vi "TEST_NT_HELPER_INT.vi"() -> ()   [LabVIEW 2023]
uses:
  <vilib>/Rock Robotics/Network Tables/NT Read Integer.vi
  <vilib>/Rock Robotics/Network Tables/NT Write Integer.vi
panel:
  out "value 2":i64
  out "value":i64
  in  "name 2":string="Test4150Val1i"
  in  "name":string="Test4150Val2i"
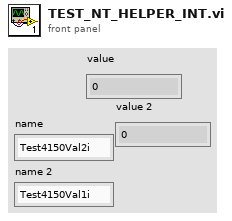
[diagram p1: front panel]
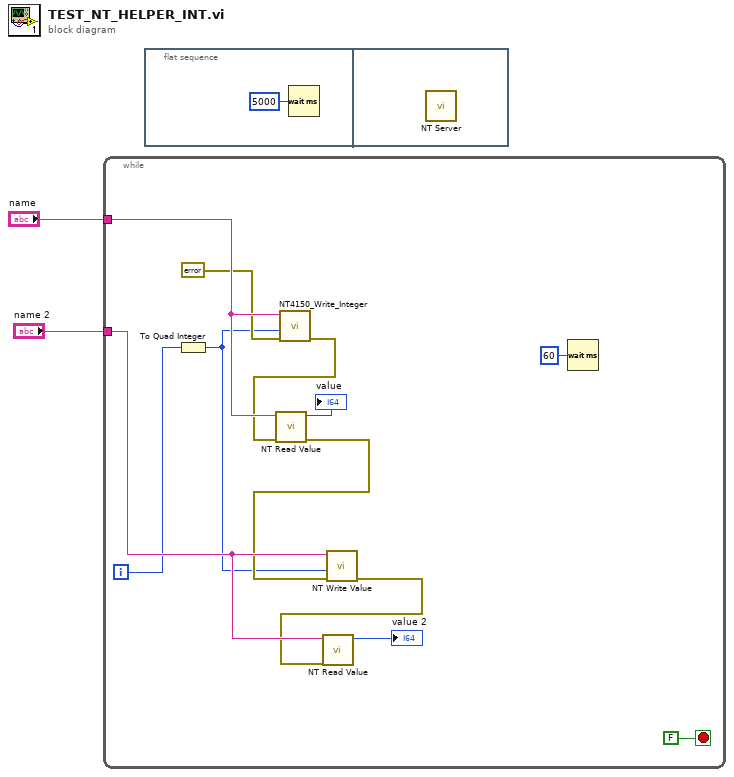
[diagram p0: block diagram]
diagram:
  n1 = while {
    tunnel: "name" -> [w14]
    tunnel: "name 2" -> [w12]
    i -> [w7]
    stop <- FALSE stop-if-true
    n2 = To Quad Integer(1:w7) -> (0:w6:i64)
    n3 = call "NT4150_Write_Integer.vi"("error in"=errorcluster {"status"=FALSE, "code"=0, "source"=""}, "value"=w6, "name"=w14) -> ("error out"=w11:errorcluster)  [unwired: 8 in]
    n4 = call-poly <vilib>:"NT Read Value.vi"("error in"=w11, "name"=w14) -> ("error out"=w10:errorcluster, "value"=→"value":i64)  [unwired: 7 in, 1 out]
    n5 = call-poly <vilib>:"NT Write Value.vi"("error in"=w10, "value"=w6, "name"=w12) -> ("error out"=w9:errorcluster)  [unwired: 8 in]
    n6 = call-poly <vilib>:"NT Read Value.vi"("error in"=w9, "name"=w12) -> ("value"=→"value 2":i64)  [unwired: 7 in, 2 out]
    n7 = Wait (ms)(milliseconds to wait=u32 60) -> ()  [unwired: 1 out]
  }
  n8 = flat-sequence {
    frame #0 {
      n9 = Wait (ms)(milliseconds to wait=u32 5000) -> ()  [unwired: 1 out]
    }
    frame #1 {
      n10 = call <vilib>:"NT Server.vi"() -> ()  [unwired: 11 in, 1 out]
    }
  }
